vi "GetReferences.vi"(8 "error in (no error)":errorcluster, 11 "3D Object in":refnum<class "3D Object.lvclass">) -> (0 "error out":errorcluster, 1 "Drawable":refnum<vi>, 2 "SceneObject":refnum<vi>, 3 "3D Object out":refnum<class "3D Object.lvclass">)   [LabVIEW 2015, in "3D Object.lvclass"]
uses:
  3D Object.lvclass
  3D Object.lvclass/3D Object.ctl
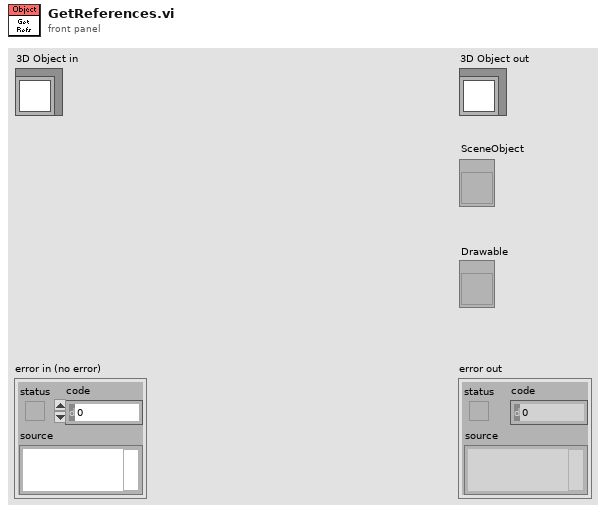
[diagram p1: front panel]
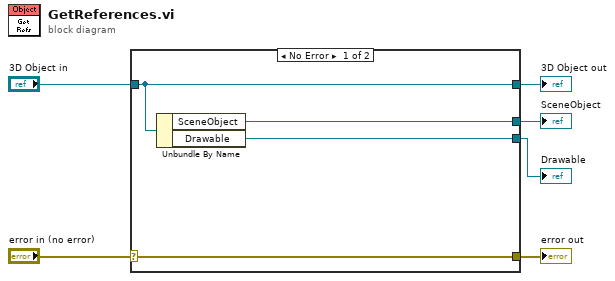
[diagram p0: block diagram]
diagram:
  n1 = case shown="No Error" "error in (no error)" {
    selector: "error in (no error)" -> [w10 w11]
    tunnel: [w10 w11] -> w5
    tunnel: [w9 w12] -> w3
    tunnel: "3D Object in" -> [w9 w12]
    tunnel: [w8 _] -> w2
    tunnel: [w7 _] -> w1
    frame No Error {
      n2 = Unbundle By Name(w9) -> ("SceneObject"=w8:refnum<vi>, "Drawable"=w7:refnum<vi>)
    }
    frame Error {
    }
  }
  "error out" <- w5
  "3D Object out" <- w3
  "SceneObject" <- w2
  "Drawable" <- w1
